vi "DAQ_channels.vi"() -> (0 "subset of DAQ channels":tag[](array[tag]), 1 "all DAQ channels":tag[](array[tag]), 2 "Channel 0":tag)   [LabVIEW 2020]
uses:
  <resource>/objmgr/daqmx.rc
panel:
  in  "# of ch.":i32=4
  in  "start ch.":i32
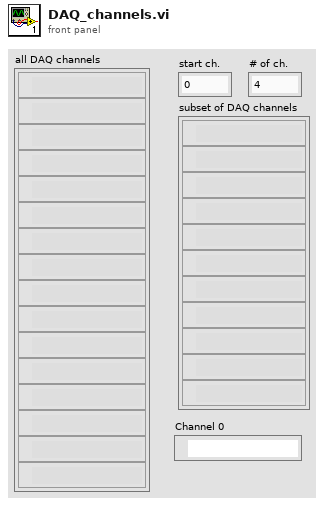
[diagram p1: front panel]
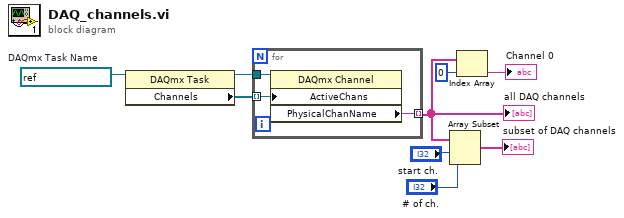
[diagram p0: block diagram]
diagram:
  w7 = refnum<k21> "VoltageTask"  # DAQmx Task Name
  n1 = property class="DAQmx Task"(reference=w7) -> (reference out=w8:refnum<k21>, "Channels"=w9:refnum<k21>[])  [unwired: 1 in, 1 out]
  n2 = for {
    tunnel: w9 -> [w12] mode=indexing
    tunnel: w8 -> [w11]
    tunnel: [w10] -> w3 mode=indexing
    n3 = property class="DAQmx Channel"(reference=w11, "ActiveChans"=w12) -> ("PhysicalChanName"=w10:tag)  [unwired: 1 in, 2 out]
  }
  "all DAQ channels" <- w3
  n4 = Array Subset(array=w3, index="start ch.", length="# of ch.") -> (→"subset of DAQ channels":tag[])
  n5 = Index Array(array=w3, index=0) -> (element=→"Channel 0":tag)
